vi "Convert Data to Offset values.vi"(0 "Messages":T1(array[cluster])) -> (13 "Offset A":sgl, 14 "OffsetHiBrdgVolt":sgl, 15 "Diff Volt A":sgl, 16 "Diff Volt B":sgl, 17 "Diff Volt C":sgl, 18 "Offset C":sgl, 19 "Offset B":sgl)   [LabVIEW 2023]
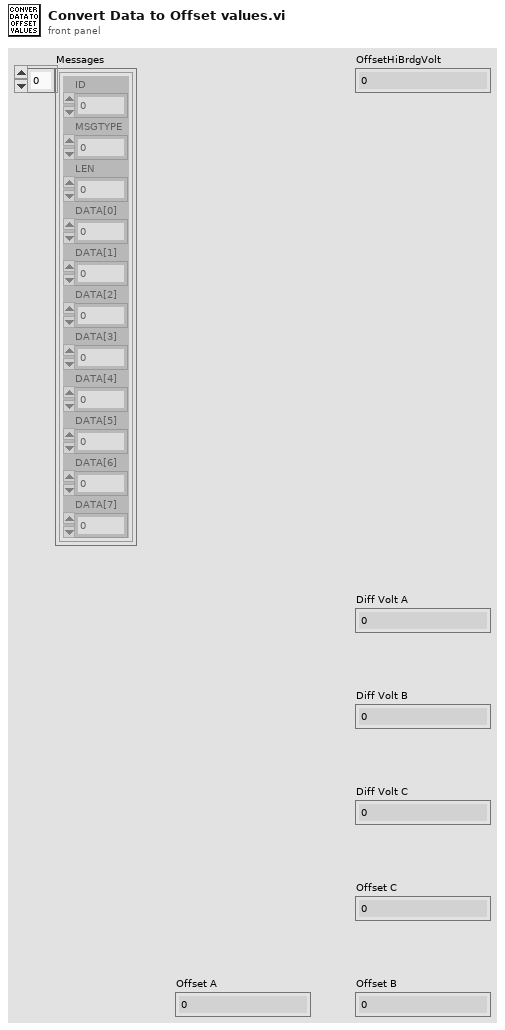
[diagram p1: front panel]
types:
  T1 = cluster{"ID":u32, "MSGTYPE":u8, "LEN":u8, "DATA[0]":u8, "DATA[1]":u8, "DATA[2]":u8, "DATA[3]":u8, "DATA[4]":u8, "DATA[5]":u8, "DATA[6]":u8, "DATA[7]":u8}[]
  T2 = cluster{"ID":u32, "MSGTYPE":u8, "LEN":u8, "DATA[0]":u8, "DATA[1]":u8, "DATA[2]":u8, "DATA[3]":u8, "DATA[4]":u8, "DATA[5]":u8, "DATA[6]":u8, "DATA[7]":u8}
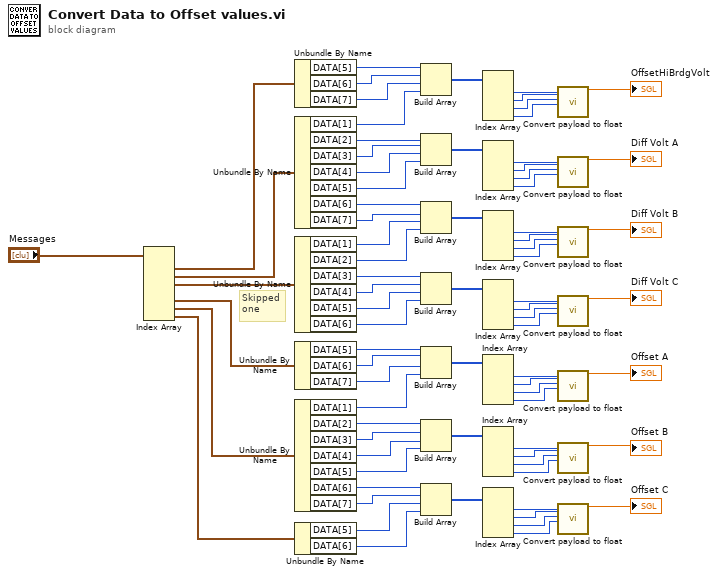
[diagram p0: block diagram]
diagram:
  # "Skipped\none"
  n1 = Index Array(array="Messages") -> (element #1=w76:T2, element #2=w75:T2, element #3=w74:T2, element #5=w73:T2, element #6=w72:T2, element #7=w71:T2)  [unwired: 7 in, 1 out]
  n2 = Unbundle By Name(w76) -> ("DATA[5]"=w70:u8, "DATA[6]"=w69:u8, "DATA[7]"=w68:u8)
  n3 = Unbundle By Name(w75) -> ("DATA[1]"=w67:u8, "DATA[2]"=w66:u8, "DATA[3]"=w65:u8, "DATA[4]"=w64:u8, "DATA[5]"=w63:u8, "DATA[6]"=w62:u8, "DATA[7]"=w61:u8)
  n4 = Unbundle By Name(w74) -> ("DATA[1]"=w60:u8, "DATA[2]"=w59:u8, "DATA[3]"=w58:u8, "DATA[4]"=w57:u8, "DATA[5]"=w56:u8, "DATA[6]"=w55:u8)
  n5 = Unbundle By Name(w73) -> ("DATA[5]"=w54:u8, "DATA[6]"=w53:u8, "DATA[7]"=w52:u8)
  n6 = Unbundle By Name(w72) -> ("DATA[1]"=w51:u8, "DATA[2]"=w50:u8, "DATA[3]"=w49:u8, "DATA[4]"=w48:u8, "DATA[5]"=w47:u8, "DATA[6]"=w46:u8, "DATA[7]"=w45:u8)
  n7 = Unbundle By Name(w71) -> ("DATA[5]"=w44:u8, "DATA[6]"=w43:u8)
  n8 = Build Array(w70, w69, w68, w67) -> (w42:u8[])
  n9 = Build Array(w66, w65, w64, w63) -> (w32:u8[])
  n10 = Build Array(w62, w61, w60, w59) -> (w27:u8[])
  n11 = Build Array(w58, w57, w56, w55) -> (w22:u8[])
  n12 = Build Array(w54, w53, w52, w51) -> (w19:u8[])
  n13 = Build Array(w50, w49, w48, w47) -> (w16:u8[])
  n14 = Build Array(w46, w45, w44, w43) -> (w13:u8[])
  n15 = Index Array(array=w42) -> (element #1=w41:u8, element #2=w40:u8, element #3=w39:u8, element #4=w38:u8)  [unwired: 4 in]
  n16 = Index Array(array=w32) -> (element #1=w33:u8, element #2=w34:u8, element #3=w35:u8, element #4=w36:u8)  [unwired: 4 in]
  n17 = Index Array(array=w27) -> (element #1=w31:u8, element #2=w30:u8, element #3=w29:u8, element #4=w28:u8)  [unwired: 4 in]
  n18 = Index Array(array=w22) -> (element #1=w23:u8, element #2=w24:u8, element #3=w25:u8, element #4=w26:u8)  [unwired: 4 in]
  n19 = Index Array(array=w19) -> (element #1=w8:u8, element #2=w7:u8, element #3=w21:u8, element #4=w20:u8)  [unwired: 4 in]
  n20 = Index Array(array=w16) -> (element #1=w10:u8, element #2=w9:u8, element #3=w17:u8, element #4=w18:u8)  [unwired: 4 in]
  n21 = Index Array(array=w13) -> (element #1=w12:u8, element #2=w11:u8, element #3=w15:u8, element #4=w14:u8)  [unwired: 4 in]
  n22 = call "Convert payload to float.vi"("Byte1"=w41, "Byte2"=w40, "Byte3"=w39, "Byte4"=w38) -> ("FloatNumber"=→"OffsetHiBrdgVolt":sgl)  [unwired: 15 in]
  n23 = call "Convert payload to float.vi"("Byte1"=w33, "Byte2"=w34, "Byte3"=w35, "Byte4"=w36) -> ("FloatNumber"=→"Diff Volt A":sgl)  [unwired: 15 in]
  n24 = call "Convert payload to float.vi"("Byte1"=w31, "Byte2"=w30, "Byte3"=w29, "Byte4"=w28) -> ("FloatNumber"=→"Diff Volt B":sgl)  [unwired: 15 in]
  n25 = call "Convert payload to float.vi"("Byte1"=w23, "Byte2"=w24, "Byte3"=w25, "Byte4"=w26) -> ("FloatNumber"=→"Diff Volt C":sgl)  [unwired: 15 in]
  n26 = call "Convert payload to float.vi"("Byte1"=w8, "Byte2"=w7, "Byte3"=w21, "Byte4"=w20) -> ("FloatNumber"=→"Offset A":sgl)  [unwired: 15 in]
  n27 = call "Convert payload to float.vi"("Byte1"=w10, "Byte2"=w9, "Byte3"=w17, "Byte4"=w18) -> ("FloatNumber"=→"Offset B":sgl)  [unwired: 15 in]
  n28 = call "Convert payload to float.vi"("Byte1"=w12, "Byte2"=w11, "Byte3"=w15, "Byte4"=w14) -> ("FloatNumber"=→"Offset C":sgl)  [unwired: 15 in]
